vi "Richtmeyer Sequence.vi"(7 "initialize?":bool=TRUE, 10 "seed":dbl=1.7320508075688772 format="%#_12g", 11 "samples":i32=128) -> (0 "error":i32, 3 "Richtmeyer Pattern":dbl[](array[numeric]) format="%#_12g")   [LabVIEW 2017, in "NI_AAL_SignalGeneration.lvlib"]
doc: "Generates quasi-random Halton or Richtmeyer sequences, which are low-discrepancy number sequences."
uses:
  <vilib>/Analysis/NI_AAL_SignalGeneration.lvlib
panel:
  # "Richtmeyer Sequence"
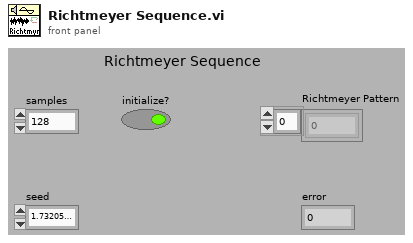
[diagram p1: front panel]
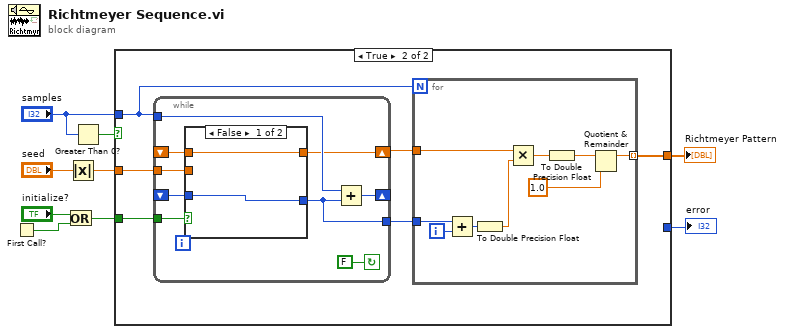
[diagram p0: block diagram]
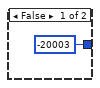
[diagram p2: hidden frame]
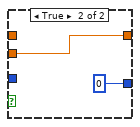
[diagram p3: hidden frame]
diagram:
  n1 = First Call?() -> (First Call?: T/F=w6:bool)
  n2 = Or(x="initialize?", y=w6) -> (x .or. y?=w5:bool)
  n3 = Absolute Value(x="seed") -> (abs(x)=w3:dbl)
  n4 = Greater Than 0?(x="samples") -> (x > 0?=w2:bool)
  n5 = case shown="True" w2 {
    tunnel: [_ w16] -> w9
    tunnel: "samples" -> [_ w15]
    tunnel: w5 -> [_ w12]
    tunnel: [-20003 _] -> w4
    tunnel: w3 -> [_ w11]
    frame False {
    }
    frame True {
      n6 = while {
        shift-right: [w23] -> _
        shift-left: _ -> [w25]
        tunnel: w11 -> [w21]
        shift-right: [w20] -> w14
        shift-left: _ -> [w19]
        tunnel: w15 -> [w22]
        tunnel: [w18] -> w13
        tunnel: w12 -> [w17]
        stop <- FALSE continue-if-true
        n7 = case shown="False" w17 {
          tunnel: w25 -> [w26 _]
          tunnel: [w26 0] -> w18
          tunnel: w21 -> [_ w28]
          tunnel: [w27 w28] -> w20
          tunnel: w19 -> [w27 _]
          frame False {
          }
          frame True {
          }
        }
        n8 = Add(x=w22, y=w18) -> (x+y=w23:i32)
      }
      n9 = for {
        N: w15 -> [_]
        tunnel: w14 -> [w36]
        tunnel: [w35] -> w16 mode=indexing
        tunnel: w13 -> [w33]
        i -> [w34]
        n10 = Add(x=w33, y=w34) -> (x+y=w32:i32)
        n11 = To Double Precision Float(number=w32) -> (double precision float=w31:dbl)
        n12 = Multiply(x=w36, y=w31) -> (x*y=w37:dbl)
        n13 = To Double Precision Float(number=w37) -> (double precision float=w30:dbl)
        n14 = Quotient & Remainder(x=w30, y=1.0) -> (x-y*floor(x/y)=w35:dbl)  [unwired: 1 out]
      }
    }
  }
  "Richtmeyer Pattern" <- w9
  "error" <- w4
